vi "Test Pass 3.vi"   [LabVIEW 2020, in "Caraya Test 19.lvlib"]
uses:
  Caraya Test 19.lvlib
  <vilib>/addons/_JKI Toolkits/Caraya/classes/Assert/Assert True.vi
  <vilib>/addons/_JKI Toolkits/Caraya/classes/Test/Test.lvclass
  <vilib>/addons/_JKI Toolkits/Caraya/classes/Assert/Assert.lvclass
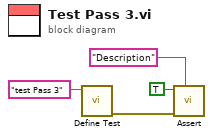
[diagram p0: block diagram]
diagram:
  n1 = call <vilib>:"Define Test.vi"("Label (VI Title)"="test Pass 3" ("Description")) -> ("error out"=w4:errorcluster)  [unwired: 10 in]
  n2 = call-poly <vilib>:"Assert.vi"("Label"="Description" ("Description"), "error in (no error)"=w4, "True?"=TRUE) -> ()  [unwired: 8 in, 1 out]
